vi "Sequence.CompleteMain.vi"(7 "Code.Main":refnum<k24>, 8 "error in (no error)":errorcluster, 10 "Sequence Channels":T1, 11 "Refs":T3) -> (0 "error out":errorcluster)   [LabVIEW 2015, in "Single Station Execution.lvlib"]
uses:
  Single Station Execution.lvlib
  Types/Sequence.MainSeqRefs.ctl
  NationalInstruments.VeriStand.RealTimeSequenceDefinitionApi
  Types/Compiled.SequenceChannels.ctl
  Types/Channel.Properties.ctl
  Main.Constants.vi
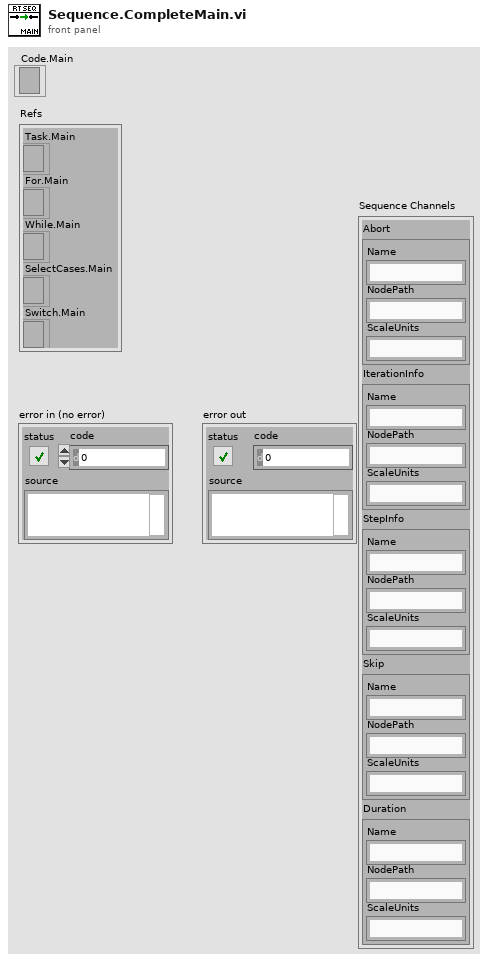
[diagram p1: front panel]
types:
  T1 = typedef "Single Station Execution.lvlib/Compiled.SequenceChannels.ctl" = cluster{"Abort":T2, "IterationInfo":T2, "StepInfo":T2, "Skip":T2, "Duration":T2}
  T2 = typedef "Single Station Execution.lvlib/Channel.Properties.ctl" = cluster{"Name":string, "NodePath":string, "ScaleUnits":string}
  T3 = typedef "Single Station Execution.lvlib/Sequence.MainSeqRefs.ctl" = cluster{"Task.Main":refnum<k24>, "For.Main":refnum<k24>, "While.Main":refnum<k24>, "SelectCases.Main":refnum<k24>, "Switch.Main":refnum<k24>}
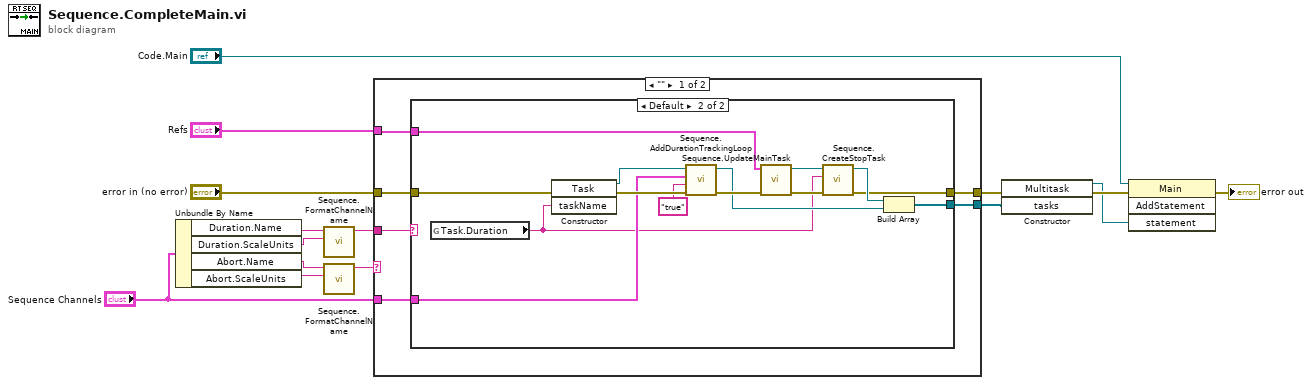
[diagram p0: block diagram]
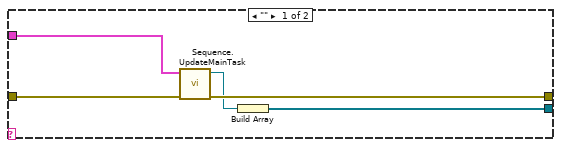
[diagram p2: hidden frame]
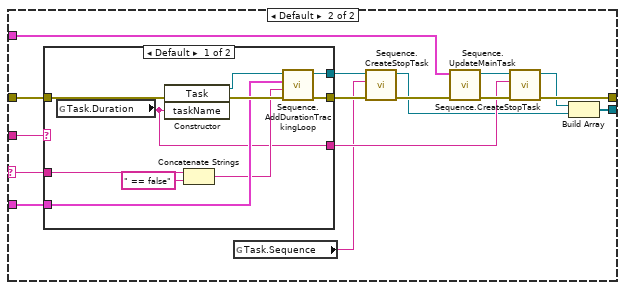
[diagram p3: hidden frame]
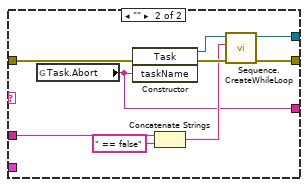
[diagram p4: hidden frame]
diagram:
  n1 = Unbundle By Name("Sequence Channels") -> ("Duration.Name"=w3:string, "Duration.ScaleUnits"=w2:string, "Abort.Name"=w6:string, "Abort.ScaleUnits"=w5:string)
  n2 = call "Sequence.FormatChannelName.vi"("ScaleUnits"=w2, "Name"=w3) -> ("ChannelName"=w1:string)  [unwired: 9 in]
  n3 = call "Sequence.FormatChannelName.vi"("ScaleUnits"=w5, "Name"=w6) -> ("ChannelName"=w7:string)  [unwired: 9 in]
  n4 = case shown="\"\"" w7 {
    selector: w7 -> [_ w55]
    tunnel: "error in (no error)" -> [w21 w56]
    tunnel: [w19 w51] -> w11
    tunnel: [w18 w54] -> w10
    tunnel: "Refs" -> [w16 w49]
    tunnel: "Sequence Channels" -> [w20 w47]
    tunnel: w1 -> [w17 w48]
    frame "" {
      n5 = case shown="Default" w17 {
        tunnel: w21 -> [w25 w40]
        tunnel: [w26 w31] -> w19
        tunnel: w20 -> [_ w37]
        tunnel: [w23 w29] -> w18
        tunnel: w16 -> [w22 w27]
        frame "" {
          n6 = call "Sequence.UpdateMainTask.vi"("error in (no error)"=w25, "Refs"=w22) -> ("error out"=w26:errorcluster, "Task.Main Ref"=w24:refnum<k24>)  [unwired: 8 in]
          n7 = Build Array(w24) -> (w23:refnum<k24>[])
        }
        frame Default {
          n8 = global read "Main.Constants.vi" "Task.Duration"() -> (w28:string)
          n9 = constructor class="Task"(error in=w40, "taskName"=w28) -> (reference out=w38:refnum<k24>, error out=w39:errorcluster)  [unwired: 2 in, 2 out]
          n10 = call "Sequence.AddDurationTrackingLoop.vi"("error in (no error)"=w39, "expressionString"="true", "Sequence Channels"=w37, ".NET Refnum in"=w38) -> ("error out"=w35:errorcluster, ".NET Refnum out"=w30:refnum<k24>)  [unwired: 6 in]
          n11 = call "Sequence.UpdateMainTask.vi"("error in (no error)"=w35, "Refs"=w27) -> ("error out"=w32:errorcluster, "Task.Main Ref"=w33:refnum<k24>)  [unwired: 8 in]
          n12 = call "Sequence.CreateStopTask.vi"("error in (no error)"=w32, "Task Name"=w28, "Task Ref"=w33) -> ("error out"=w31:errorcluster, ".NET Refnum out"=w34:refnum<k24>)  [unwired: 7 in]
          n13 = Build Array(w34, w30) -> (w29:refnum<k24>[])
        }
      }
    }
    frame Default {
      n14 = case shown="Default" w48 {
        tunnel: w56 -> [w64 w75]
        tunnel: w55 -> [w61 w72]
        tunnel: [w58 w67] -> w44
        tunnel: w47 -> [w63 _]
        tunnel: [w59 w69] -> w46
        tunnel: [w57 w68] -> w43
        frame Default {
          n15 = global read "Main.Constants.vi" "Task.Duration"() -> (w59:string)
          n16 = constructor class="Task"(error in=w64, "taskName"=w59) -> (reference out=w65:refnum<k24>, error out=w66:errorcluster)  [unwired: 2 in, 2 out]
          n17 = Concatenate Strings(w61, " == false" ("string")) -> (w60:string)
          n18 = call "Sequence.AddDurationTrackingLoop.vi"("error in (no error)"=w66, "expressionString"=w60, "Sequence Channels"=w63, ".NET Refnum in"=w65) -> ("error out"=w58:errorcluster, ".NET Refnum out"=w57:refnum<k24>)  [unwired: 6 in]
        }
        frame "" {
          n19 = global read "Main.Constants.vi" "Task.Abort"() -> (w69:string)
          n20 = constructor class="Task"(error in=w75, "taskName"=w69) -> (reference out=w74:refnum<k24>, error out=w73:errorcluster)  [unwired: 2 in, 2 out]
          n21 = Concatenate Strings(w72, " == false" ("string")) -> (w70:string)
          n22 = call "Sequence.CreateWhileLoop.vi"("error in (no error)"=w73, "Expression"=w70, "Task Ref"=w74) -> ("error out"=w67:errorcluster, "Task Ref out"=w68:refnum<k24>)  [unwired: 7 in]
        }
      }
      n23 = global read "Main.Constants.vi" "Task.Sequence"() -> (w41:string)
      n24 = call "Sequence.CreateStopTask.vi"("error in (no error)"=w44, "Task Name"=w41, "Task Ref"=w43) -> ("error out"=w45:errorcluster, ".NET Refnum out"=w42:refnum<k24>)  [unwired: 7 in]
      n25 = call "Sequence.UpdateMainTask.vi"("error in (no error)"=w45, "Refs"=w49) -> ("error out"=w52:errorcluster, "Task.Main Ref"=w53:refnum<k24>)  [unwired: 8 in]
      n26 = call "Sequence.CreateStopTask.vi"("error in (no error)"=w52, "Task Name"=w46, "Task Ref"=w53) -> ("error out"=w51:errorcluster, ".NET Refnum out"=w50:refnum<k24>)  [unwired: 7 in]
      n27 = Build Array(w50, w42) -> (w54:refnum<k24>[])
    }
  }
  n28 = constructor class="Multitask"(error in=w11, "tasks"=w10) -> (reference out=w13:refnum<k24>, error out=w14:errorcluster)  [unwired: 2 in, 2 out]
  n29 = invoke class="Main" method="AddStatement"(reference="Code.Main", error in=w14, "statement"=w13) -> (error out=→"error out":errorcluster)  [unwired: 1 in, 3 out]
